vi "Galvo Error.vi"(8 "error in (no error)":errorcluster) -> (0 "error out":errorcluster)   [LabVIEW 2014]
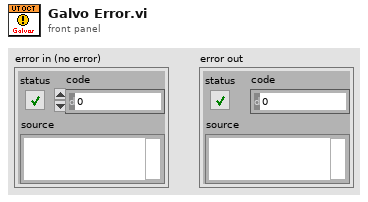
[diagram p1: front panel]
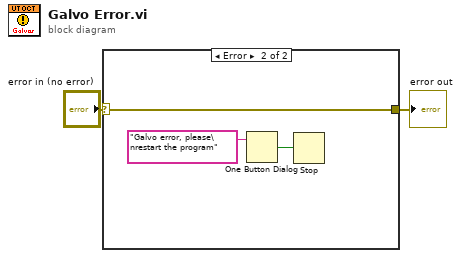
[diagram p0: block diagram]
diagram:
  n1 = case shown="Error" "error in (no error)" {
    selector: "error in (no error)" -> [w3 w4]
    tunnel: [w3 w4] -> w2
    frame No Error {
    }
    frame Error {
      n2 = One Button Dialog(message="Galvo error, please\nrestart the program") -> (true=w5:bool)  [unwired: 1 in]
      n3 = Stop(stop? (T)=w5) -> ()
    }
  }
  "error out" <- w2
